vi "TestPFGVRequests.vi"() -> (0 "error out":errorcluster, 2 "Pass":bool)   [LabVIEW 2015]
uses:
  TypeDef/PersonnelActions.ctl
  LVClasses/Flags/Flags.lvclass
  LVClasses/Room/Room.lvclass
panel:
  out "Add Request 2":string
  out "Read Request 2":string
  out "Remove Request":string
  out "Add Request 1":string
  out "Read Personnel 3":string
  out "Read Personnel":string
  out "Read Personnel 2":string
  out "Read Requests 1":string
  in  "PUID":string="d1"
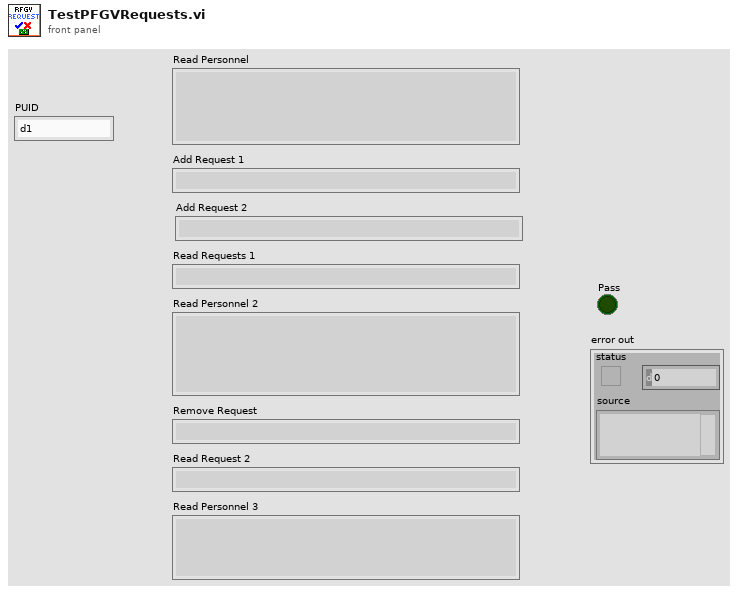
[diagram p1: front panel]
types:
  T1 = typedef "PersonnelActions.ctl" = enum16{"Init", "Read Personnel", "Add Personnel", "Remove Personnel", "Read Name", "Write Name", "Read Role", "Write Role", "Read Requests", "Add Requests", "Remove Requests", "Read PUIDs"}
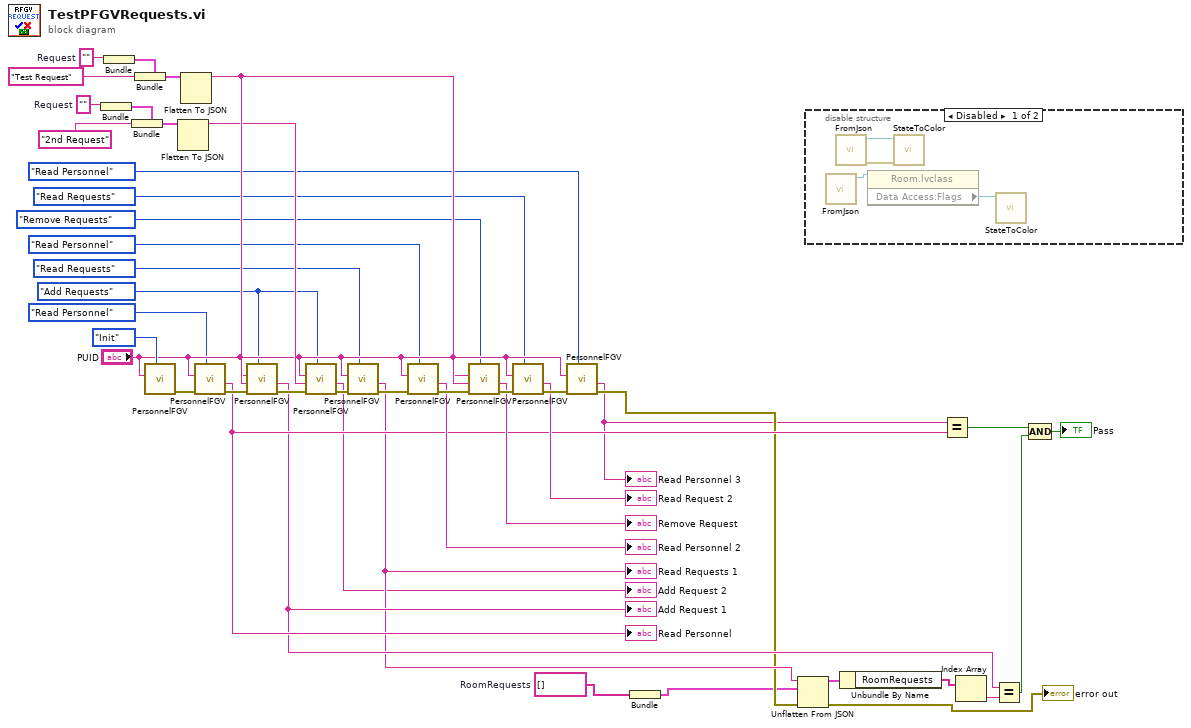
[diagram p0: block diagram]
diagram:
  w2 = PersonnelActions."Add Requests" ("Actions")
  w17 = ""  # Request
  w14 = string[] []  # RoomRequests
  w39 = ""  # Request
  n1 = Bundle("Request"=w17) -> (w18:cluster{"Request":string})  [unwired: 1 in]
  n2 = Bundle("Request"=w39) -> (w38:cluster{"Request":string})  [unwired: 1 in]
  n3 = Bundle(cluster=w18, "Request"="2nd Request" ("Request 2")) -> (w19:cluster{"Request":string})
  n4 = Bundle(cluster=w38, "Request"="Test Request") -> (w37:cluster{"Request":string})
  n5 = call "PersonnelFGV.vi"("Actions"=PersonnelActions."Init", "PUID"="PUID") -> ("error out"=w45:errorcluster)  [unwired: 8 in, 1 out]
  n6 = Flatten To JSON(anything=w19) -> (JSON string=w16:string)  [unwired: 2 in, 1 out]
  n7 = Flatten To JSON(anything=w37) -> (JSON string=w34:string)  [unwired: 2 in, 1 out]
  n8 = call "PersonnelFGV.vi"("Actions"=PersonnelActions."Read Personnel", "error in (no error)"=w45, "PUID"="PUID") -> ("error out"=w44:errorcluster, "Data Out"=w31:string)  [unwired: 7 in]
  "Read Personnel" <- w31
  n9 = call "PersonnelFGV.vi"("Actions"=w2, "error in (no error)"=w44, "Data In"=w34, "PUID"="PUID") -> ("error out"=w40:errorcluster, "Data Out"=w27:string)  [unwired: 6 in]
  "Add Request 1" <- w27
  n10 = call "PersonnelFGV.vi"("Actions"=w2, "error in (no error)"=w40, "Data In"=w16, "PUID"="PUID") -> ("error out"=w21:errorcluster, "Data Out"=→"Add Request 2":string)  [unwired: 6 in]
  n11 = call "PersonnelFGV.vi"("Actions"=PersonnelActions."Read Requests", "error in (no error)"=w21, "PUID"="PUID") -> ("error out"=w43:errorcluster, "Data Out"=w26:string)  [unwired: 7 in]
  "Read Requests 1" <- w26
  n12 = call "PersonnelFGV.vi"("Actions"=PersonnelActions."Read Personnel", "error in (no error)"=w43, "PUID"="PUID") -> ("error out"=w42:errorcluster, "Data Out"=→"Read Personnel 2":string)  [unwired: 7 in]
  n13 = call "PersonnelFGV.vi"("Actions"=PersonnelActions."Remove Requests", "error in (no error)"=w42, "Data In"=w34, "PUID"="PUID") -> ("error out"=w36:errorcluster, "Data Out"=→"Remove Request":string)  [unwired: 6 in]
  n14 = call "PersonnelFGV.vi"("Actions"=PersonnelActions."Read Requests", "error in (no error)"=w36, "PUID"="PUID") -> ("error out"=w35:errorcluster, "Data Out"=→"Read Request 2":string)  [unwired: 7 in]
  n15 = call "PersonnelFGV.vi"("Actions"=PersonnelActions."Read Personnel", "error in (no error)"=w35, "PUID"="PUID") -> ("error out"=w23:errorcluster, "Data Out"=w10:string)  [unwired: 7 in]
  "Read Personnel 3" <- w10
  n16 = Bundle("RoomRequests"=w14) -> (w13:cluster{"RoomRequests":string[]})  [unwired: 1 in]
  n17 = Unflatten From JSON(JSON string=w26, type and defaults=w13, error in (no error)=w23) -> (value=w12:cluster{"RoomRequests":string[]}, error out=→"error out":errorcluster)  [unwired: 4 in]
  n18 = disable-structure shown="Disabled" {
    frame Disabled {
      n19 = call "FromJson.vi"() -> ("Room out"=w47:refnum<class "Room.lvclass">)  [unwired: 10 in, 1 out]
      n20 = call "FromJson.vi"() -> ("error out"=w49:errorcluster, "Flags out"=w48:refnum<class "Flags.lvclass">)  [unwired: 10 in]
      n21 = property class="Room.lvclass"(reference=w47) -> ("Data Access:Flags"=w46:refnum<class "Flags.lvclass">)  [unwired: 1 in, 2 out]
      n22 = call "StateToColor.vi"("error in (no error)"=w49, "Flags in"=w48) -> ()  [unwired: 7 in, 3 out]
      n23 = call "StateToColor.vi"("Flags in"=w46) -> ()  [unwired: 8 in, 3 out]
    }
    frame Enabled {
    }
  }
  n24 = Unbundle By Name(w12) -> ("RoomRequests"=w11:string[])
  n25 = Equal?(x=w10, y=w31) -> (x = y?=w30:bool)
  n26 = Index Array(array=w11) -> (element=w24:string)  [unwired: 1 in]
  n27 = Equal?(x=w27, y=w24) -> (x = y?=w28:bool)
  n28 = Compound Arithmetic op=AND(w30, w28) -> (→"Pass":bool)
